vi "Calc Roll.vi"(10 "Position":dbl) -> (2 "Roll":dbl)   [LabVIEW 2014]
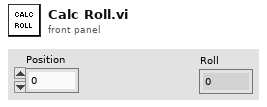
[diagram p1: front panel]
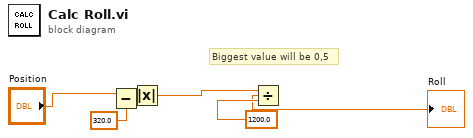
[diagram p0: block diagram]
diagram:
  # "Biggest value will be 0,5"
  n1 = Subtract(x="Position", y=320.0) -> (x-y=w4:dbl)
  n2 = Absolute Value(x=w4) -> (abs(x)=w3:dbl)
  n3 = Divide(x=w3, y=1200.0) -> (x/y=→"Roll":dbl)
